vi "Set Laser Power.vi"(8 "error in (no error)":errorcluster, 9 "Power":dbl, 10 "Wavelength":u16, 11 "Laser Quantum in":refnum<class "Laser Quantum.lvclass">) -> (0 "error out":errorcluster, 3 "Laser Quantum out":refnum<class "Laser Quantum.lvclass">)   [LabVIEW 2018, in "Laser Quantum.lvlib" / "Laser Quantum.lvclass"]
uses:
  Laser Quantum.lvclass
  Laser Quantum.lvclass/Laser Quantum.ctl
  Laser Quantum.lvlib
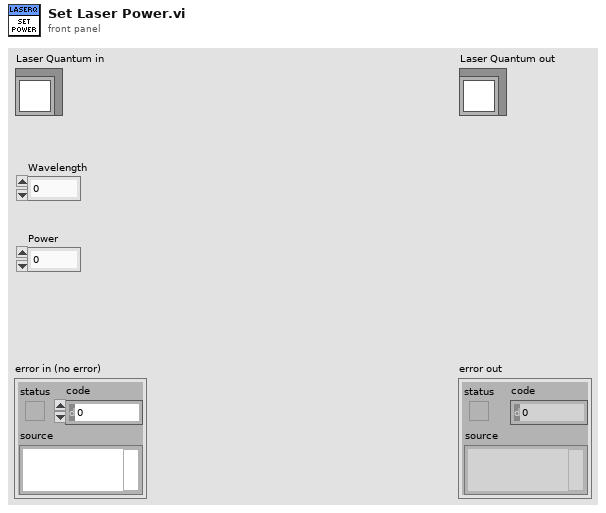
[diagram p1: front panel]
types:
  T1 = enum16{"Disable", "Laser Quantum", "Coherent OBIS", "PRM1-Z8"}
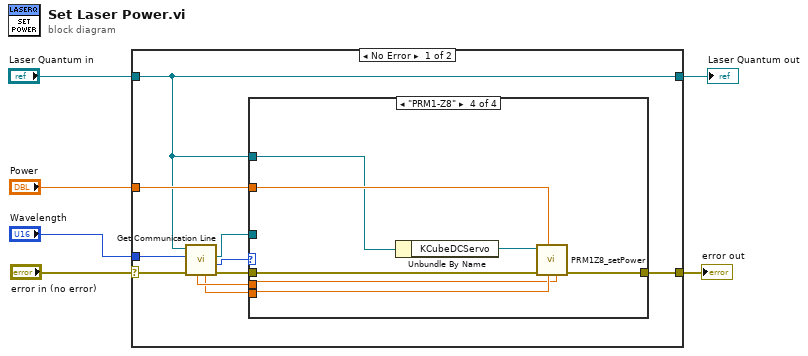
[diagram p0: block diagram]
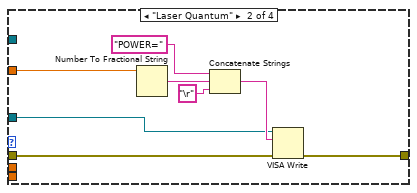
[diagram p3: hidden frame]
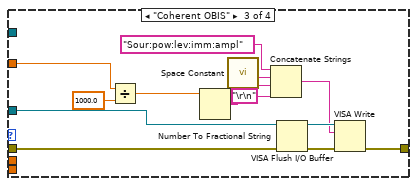
[diagram p4: hidden frame]
diagram:
  n1 = case shown="No Error" "error in (no error)" {
    selector: "error in (no error)" -> [w13 w47]
    tunnel: [w15 w47] -> w5
    tunnel: [w7 w46] -> w3
    tunnel: "Laser Quantum in" -> [w7 w46]
    tunnel: "Wavelength" -> [w14 _]
    tunnel: "Power" -> [w16 _]
    frame No Error {
      n2 = call-dynamic "Get Communication Line.vi"("error in (no error)"=w13, "Wavelength"=w14, "Laser Quantum in"=w7) -> ("error out"=w12:errorcluster, "Laser Type"=w10:T1, "Serial Port"=w11:refnum<visa-resource-name>, "Polarizer Theta Zero"=w8:dbl, "Polarizer Amplitude"=w9:dbl)  [unwired: 3 in, 1 out]
      n3 = case shown="\"PRM1-Z8\"" w10 {
        tunnel: w12 -> [w17 w19 w28 w42]
        tunnel: w16 -> [_ w25 w29 w43]
        tunnel: [w17 w21 w27 w45] -> w15
        tunnel: w11 -> [_ w18 w26 _]
        tunnel: w9 -> [_ _ _ w41]
        tunnel: w8 -> [_ _ _ w40]
        tunnel: w7 -> [_ _ _ w39]
        frame "Disable", Default {
        }
        frame "Laser Quantum" {
          n4 = Number To Fractional String(number=w25) -> (F-format string=w23:string)  [unwired: 3 in]
          n5 = Concatenate Strings("POWER=" ("write buffer"), w23, "\r" ("string")) -> (w22:string)
          n6 = VISA Write(VISA resource name=w18, write buffer=w22, error in (no error)=w19) -> (error out=w21:errorcluster)  [unwired: 2 out]
        }
        frame "Coherent OBIS" {
          n7 = Divide(x=w29, y=1000.0) -> (x/y=w34:dbl)
          n8 = Number To Fractional String(number=w34) -> (F-format string=w36:string)  [unwired: 3 in]
          n9 = call <vilib>:"Space Constant.vi"() -> ("String"=w35:string)
          n10 = Concatenate Strings("Sour:pow:lev:imm:ampl" ("write buffer"), w35, w36, "\r\n") -> (w33:string)
          n11 = VISA Flush I/O Buffer(VISA resource name=w26, error in (no error)=w28) -> (VISA resource name out=w37:refnum<visa-resource-name>, error out=w38:errorcluster)  [unwired: 1 in]
          n12 = VISA Write(VISA resource name=w37, write buffer=w33, error in (no error)=w38) -> (error out=w27:errorcluster)  [unwired: 2 out]
        }
        frame "PRM1-Z8" {
          n13 = Unbundle By Name(w39) -> ("KCubeDCServo"=w44:refnum<k24>)
          n14 = call "PRM1Z8_setPower.vi"("zero angle"=w40, "max power"=w41, "Target Power"=w43, "error in (no error)"=w42, "reference"=w44) -> ("error out"=w45:errorcluster)  [unwired: 5 in, 1 out]
        }
      }
    }
    frame Error {
    }
  }
  "error out" <- w5
  "Laser Quantum out" <- w3
